vi "Read Value.vi"(8 "error in (no error)":errorcluster caption="entrée d'erreur (pas d'erreur)", 11 "DAQmxTaskCounterDigital_Emulate en entrée":refnum<class "DAQmxTaskCounterDigital_Emulate.lvclass">) -> (0 "error out":errorcluster caption="sortie d'erreur", 1 "Data":bool, 2 "Data string":string, 3 "DAQmxTaskCounterDigital_Emulate en sortie":refnum<class "DAQmxTaskCounterDigital_Emulate.lvclass">)   [LabVIEW 2020, in "DAQmxTaskCounterDigital_Emulate.lvclass"]
uses:
  DAQmxTaskCounterDigital_Emulate.lvclass
  dependecies/globalVarII.vi
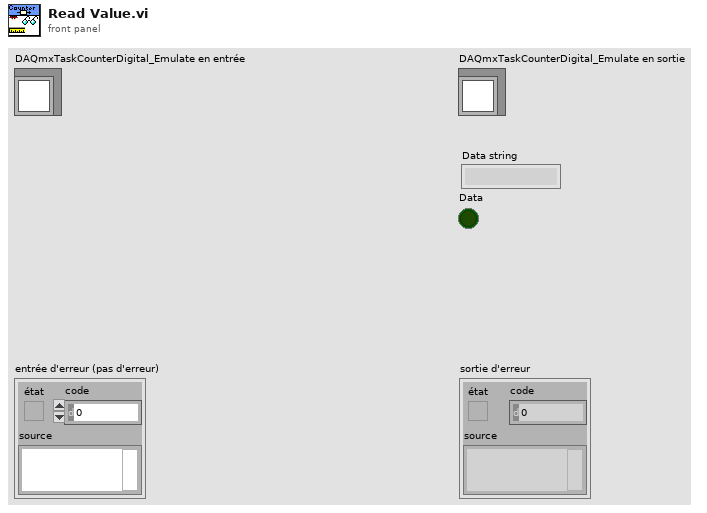
[diagram p1: front panel]
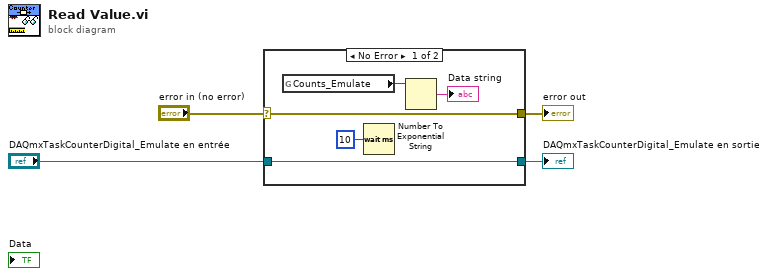
[diagram p0: block diagram]
diagram:
  n1 = case shown="No Error" "error in (no error)" {
    selector: "error in (no error)" -> [w6 w11]
    tunnel: [w6 w11] -> w3
    tunnel: [w7 w10] -> w2
    tunnel: "DAQmxTaskCounterDigital_Emulate en entrée" -> [w7 w10]
    frame No Error {
      n2 = global read "globalVarII.vi" "Counts_Emulate"() -> (w8:i64)
      n3 = Wait (ms)(milliseconds to wait=u32 10) -> ()  [unwired: 1 out]
      n4 = Number To Exponential String(number=w8) -> (E-format string=→"Data string":string)  [unwired: 3 in]
    }
    frame Error {
    }
  }
  "error out" <- w3
  "DAQmxTaskCounterDigital_Emulate en sortie" <- w2
